vi "Not A Telnet Connection.vi"() -> (0 "not a telnet connection":T1)   [LabVIEW 2014]
uses:
  Telnet Session.ctl
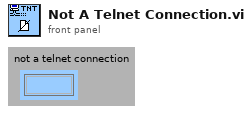
[diagram p1: front panel]
types:
  T1 = typedef "Telnet Session.ctl" = refnum<k1>
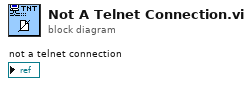
[diagram p0: block diagram]
diagram:
